vi "Module Loop.vi"(8 "error in (no error)":errorcluster, 11 "ValveControlModule in":refnum<class "ValveControlModule.lvclass">) -> (0 "error out":errorcluster, 3 "ValveControlModule out":refnum<class "ValveControlModule.lvclass">)   [LabVIEW 2020, in "VolatusControl.lvlib" / "ValveControlModule.lvclass"]
uses:
  ValveControlModule.lvclass
  C:/dev/lv20CE/relink/lv-volatus/Volatus/Module/Module.lvclass
  Volatus/Module/Module.lvclass
  Volatus/Module/Module.lvclass/Module.ctl
  messages/CmdDigital/Class/Msg.lvclass
  C:/dev/lv20CE/relink/lv-protoc/LV-Proto/Message/Message.lvclass
  messages/CmdDigital/Class/Msg.lvclass/Msg.ctl
  Volatus/MessageQ/MessageQ.lvclass/MessageQ.ctl
  messages/CmdDigital/Data.ctl
  ValveControlModule.lvclass/ValveControlModule.ctl
  messages/CmdDigitalMultiple/Data.ctl
  messages/CmdAnalog/Class/Msg.lvclass
  messages/CmdAnalog/Class/Msg.lvclass/Msg.ctl
  messages/CmdAnalog/Data.ctl
  Volatus/Module/Self Q.vi
  Volatus/MessageQ/Send.vi
  lv-vecto/Vecto/Group/Group.lvclass
  C:/dev/lv20CE/relink/lv-vecto/Vecto/GroupAbstract/GroupAbstract.lvclass
  Valve/ValveControl.lvclass
  messages/CmdDigital/CmdDigital.lvlib
  messages/CmdDigitalMultiple/CmdDigitalMultiple.lvlib
  messages/CmdAnalog/CmdAnalog.lvlib
  lv-vecto/Vecto/GroupAbstract/GroupAbstract.lvclass
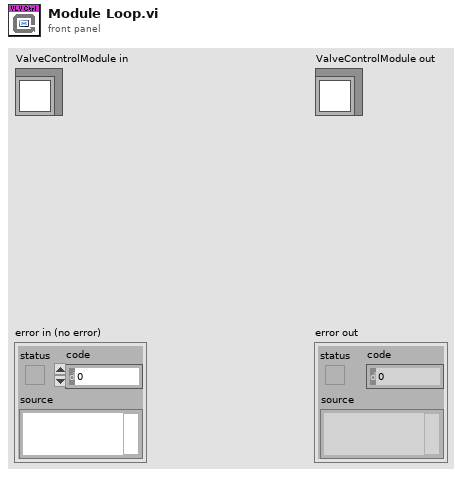
[diagram p1: front panel]
types:
  T1 = typedef "CmdDigital.lvlib/Data.ctl" = cluster{"channel":string, "value":bool}
  T2 = typedef "CmdDigitalMultiple.lvlib/Data.ctl" = cluster{"values":T1[]}
  T3 = typedef "CmdAnalog.lvlib/Data.ctl" = cluster{"channel":string, "value":dbl}
  T4 = map{string, refnum<class "ValveControl.lvclass">}
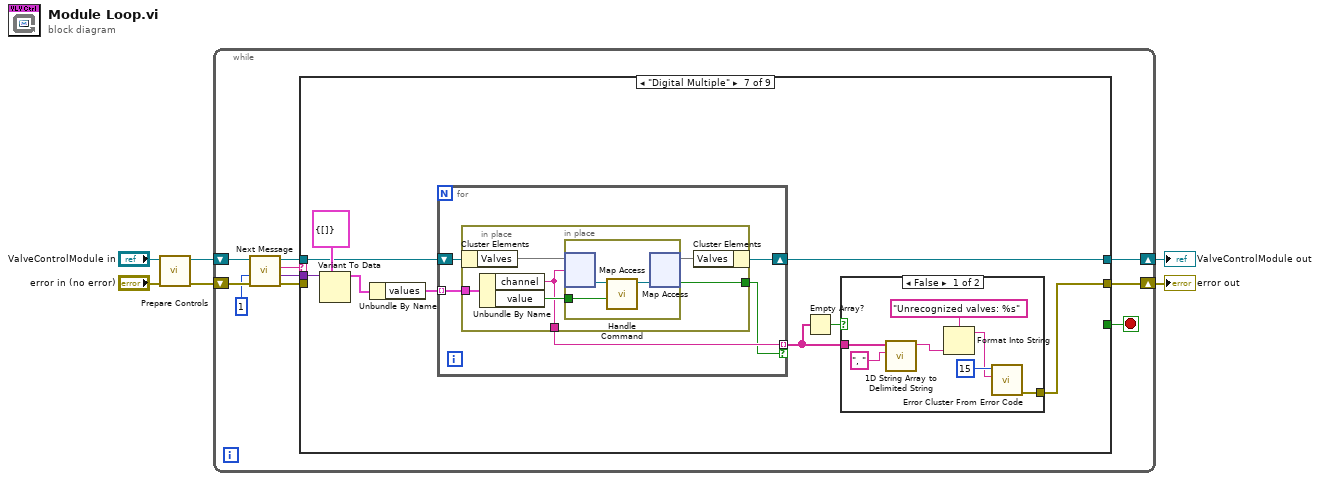
[diagram p0: block diagram]
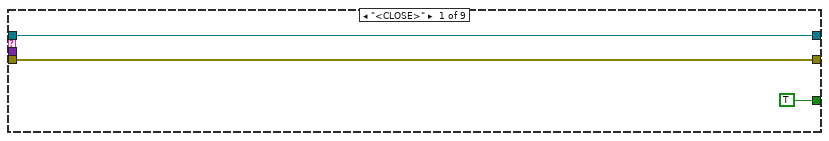
[diagram p2: hidden frame]
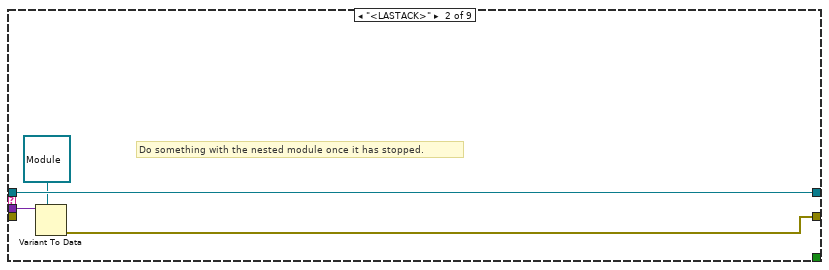
[diagram p3: hidden frame]
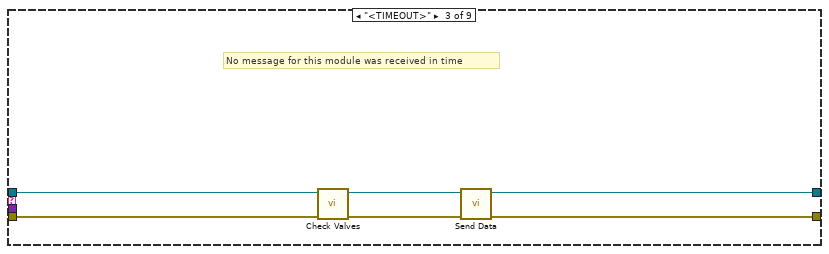
[diagram p4: hidden frame]
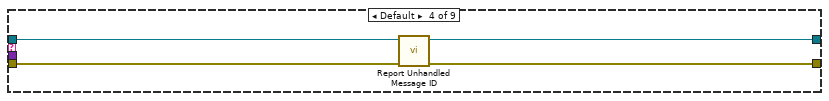
[diagram p5: hidden frame]
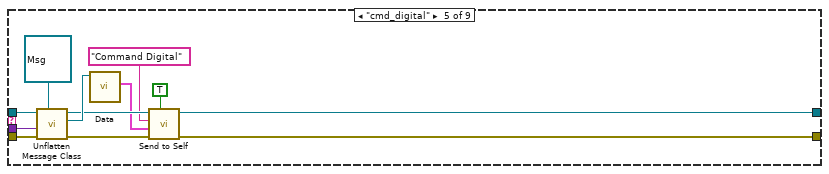
[diagram p6: hidden frame]
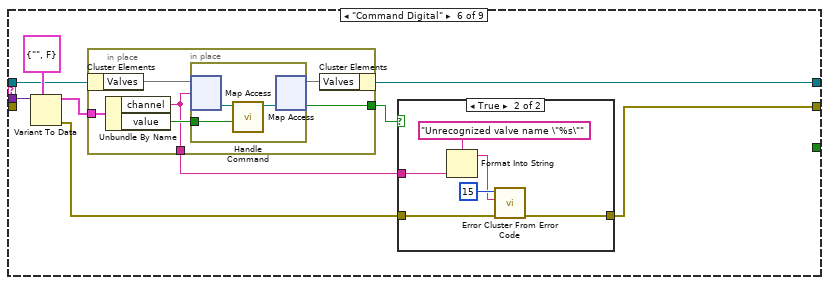
[diagram p7: hidden frame]
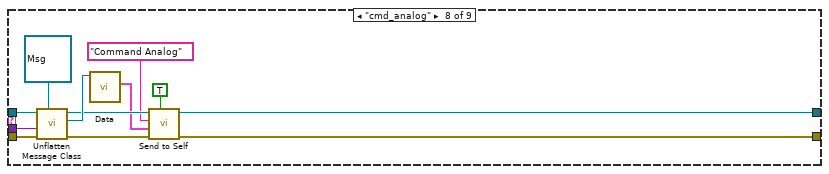
[diagram p10: hidden frame]
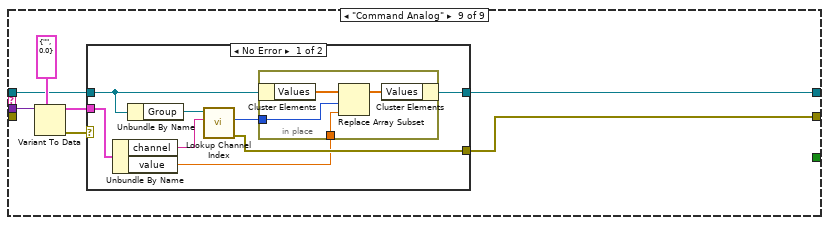
[diagram p11: hidden frame]
diagram:
  n1 = call "Prepare Controls.vi"("error in (no error)"="error in (no error)", "ValveControlModule in"="ValveControlModule in") -> ("error out"=w3:errorcluster, "ValveControlModule out"=w1:refnum<class "ValveControlModule.lvclass">)  [unwired: 8 in]
  n2 = while {
    shift-right: [w11] -> w5
    shift-left: w1 -> [w16]
    shift-right: [w10] -> w4
    shift-left: w3 -> [w15]
    stop <- w9 stop-if-true
    n3 = call "Next Message.vi"("error in (no error)"=w15, "Timeout ms (-1)"=1, "Module in"=w16) -> ("error out"=w14:errorcluster, "Data"=w8:variant, "ID"=w13:string, "Module out"=w12:refnum<class "ValveControlModule.lvclass">)  [unwired: 5 in]
    n4 = case shown="\"Digital Multiple\"" w13 {
      tunnel: w14 -> [w17 _ w29 w33 w44 _ _ w111 _]
      tunnel: w12 -> [w18 w23 w27 w31 w45 w52 w77 w112 w115]
      tunnel: [w18 w23 w24 w30 w36 w50 w76 w103 w113] -> w11
      tunnel: [w17 w20 w26 w32 w34 w46 w75 w101 w114] -> w10
      tunnel: [TRUE _ _ _ _ _ _ _ _] -> w9
      tunnel: w8 -> [_ w22 _ _ w43 w54 w79 w110 w119]
      frame "<CLOSE>" {
      }
      frame "<LASTACK>" {
        # "Do something with the nested module once it has stopped."
        n5 = Variant To Data(type=refnum<class "Module.lvclass"> refnum ("Volatus:Module"), Variant=w22) -> (error out=w20:errorcluster)  [unwired: 1 in, 1 out]
      }
      frame "<TIMEOUT>" {
        # "No message for this module was received in time"
        n6 = call "Check Valves.vi"("error in (no error)"=w29, "ValveControlModule in"=w27) -> ("error out"=w28:errorcluster, "ValveControlModule out"=w25:refnum<class "ValveControlModule.lvclass">)  [unwired: 8 in]
        n7 = call "Send Data.vi"("error in (no error)"=w28, "ValveControlModule in"=w25) -> ("error out"=w26:errorcluster, "ValveControlModule out"=w24:refnum<class "ValveControlModule.lvclass">)  [unwired: 8 in]
      }
      frame Default {
        n8 = call "Report Unhandled Message ID.vi"("error in (no error)"=w33, "Module in"=w31) -> ("error out"=w32:errorcluster, "Module out"=w30:refnum<class "ValveControlModule.lvclass">)  [unwired: 8 in]
      }
      frame "cmd_digital" {
        n9 = call "Unflatten Message Class.vi"("Message Type"=refnum<class "Msg.lvclass"> refnum ("CmdDigital.lvlib:Msg.lvclass"), "error in (no error)"=w44, "Data"=w43, "Module in"=w45) -> ("error out"=w39:errorcluster, "Message"=w41:refnum<class "Msg.lvclass">, "Module out"=w40:refnum<class "ValveControlModule.lvclass">)  [unwired: 4 in, 1 out]
        n10 = call "Data.vi"("PB Msg Template in"=w41) -> ("Data"=w37:T1)  [unwired: 8 in, 2 out]
        n11 = call "Send to Self.vi"("High Priority (F)"=TRUE, "error in (no error)"=w39, "Data"=w37, "Message ID"="Command Digital", "Module in"=w40) -> ("error out"=w34:errorcluster, "Module out"=w36:refnum<class "ValveControlModule.lvclass">)  [unwired: 5 in]
      }
      frame "Command Digital" {
        n12 = Variant To Data(type=T1 {"channel"="", "value"=FALSE} ("CmdDigital"), Variant=w54) -> (data=w51:T1, error out=w47:errorcluster)  [unwired: 1 in]
        n13 = in-place {
          in-place-border: w51 -> [w67]
          in-place-border: [w63] -> w49
          in-place-border: [w62] -> w48
          n14 = in-place-cluster #1(w52) -> ("Valves"=w66:T4)
          n15 = Unbundle By Name(w67) -> ("channel"=w62:string, "value"=w65:bool)
          n16 = in-place {
            in-place-border: w65 -> [w69]
            n17 = in-place-map #2(w66, w62) -> (w70:refnum<class "ValveControl.lvclass">)  [unwired: 1 in, 1 out]
            n18 = call-dynamic "Handle Command.vi"("Value"=w69, "Valve in"=w70) -> ("Valve out"=w68:refnum<class "ValveControl.lvclass">)  [unwired: 8 in, 1 out]
            n19 = in-place-map #2(w68) -> (w64:T4, w63:bool)  [unwired: 1 in, 1 out]
          }
          n20 = in-place-cluster #1("Valves"=w64) -> (w50:refnum<class "ValveControlModule.lvclass">)
        }
        n21 = case shown="True" w49 {
          tunnel: w48 -> [_ w61]
          tunnel: w47 -> [w55 w57]
          tunnel: [w55 w56] -> w46
          frame False {
          }
          frame True {
            n22 = Format Into String(format string="Unrecognized valve name \"%s\"", w61) -> (resulting string=w58:string)  [unwired: 2 in, 1 out]
            n23 = call <vilib>:"Error Cluster From Error Code.vi"("error in (no error)"=w57, "error message (\"\")"=w58, "error code (0)"=15) -> ("error out"=w56:errorcluster)  [unwired: 6 in]
          }
        }
      }
      frame "Digital Multiple" {
        n24 = Variant To Data(type=T2 {"values"=[]} ("CmdDigitalMultiple"), Variant=w79) -> (data=w74:T2)  [unwired: 1 in, 1 out]
        n25 = Unbundle By Name(w74) -> ("values"=w73:T1[])
        n26 = for {
          shift-right: [w83] -> w76
          shift-left: w77 -> [w84]
          tunnel: w73 -> [w82] mode=indexing
          tunnel: [w81] -> w71 mode=indexing if=w80
          n27 = in-place {
            in-place-border: [w87] -> w80
            in-place-border: [w85] -> w81
            in-place-border: w82 -> [w86]
            n28 = in-place-cluster #3(w84) -> ("Valves"=w90:T4)
            n29 = Unbundle By Name(w86) -> ("channel"=w85:string, "value"=w89:bool)
            n30 = in-place {
              in-place-border: w89 -> [w91]
              n31 = in-place-map #4(w90, w85) -> (w93:refnum<class "ValveControl.lvclass">)  [unwired: 1 in, 1 out]
              n32 = call-dynamic "Handle Command.vi"("Value"=w91, "Valve in"=w93) -> ("Valve out"=w92:refnum<class "ValveControl.lvclass">)  [unwired: 8 in, 1 out]
              n33 = in-place-map #4(w92) -> (w88:T4, w87:bool)  [unwired: 1 in, 1 out]
            }
            n34 = in-place-cluster #3("Valves"=w88) -> (w83:refnum<class "ValveControlModule.lvclass">)
          }
        }
        n35 = Empty Array?(array=w71) -> (empty?=w72:bool)
        n36 = case shown="False" w72 {
          tunnel: [w97 _] -> w75
          tunnel: w71 -> [w96 _]
          frame False {
            n37 = call <vilib>:"1D String Array to Delimited String.vi"("delimiter"=", ", "string array"=w96) -> ("delimited string"=w94:string)  [unwired: 9 in]
            n38 = Format Into String(format string="Unrecognized valves: %s", w94) -> (resulting string=w98:string)  [unwired: 2 in, 1 out]
            n39 = call <vilib>:"Error Cluster From Error Code.vi"("error message (\"\")"=w98, "error code (0)"=15) -> ("error out"=w97:errorcluster)  [unwired: 7 in]
          }
          frame True {
          }
        }
      }
      frame "cmd_analog" {
        n40 = call "Unflatten Message Class.vi"("Message Type"=refnum<class "Msg.lvclass"> refnum ("CmdAnalog.lvlib:Msg.lvclass"), "error in (no error)"=w111, "Data"=w110, "Module in"=w112) -> ("error out"=w106:errorcluster, "Message"=w108:refnum<class "Msg.lvclass">, "Module out"=w107:refnum<class "ValveControlModule.lvclass">)  [unwired: 4 in, 1 out]
        n41 = call "Data.vi"("PB Msg Template in"=w108) -> ("Data"=w104:T3)  [unwired: 8 in, 2 out]
        n42 = call "Send to Self.vi"("High Priority (F)"=TRUE, "error in (no error)"=w106, "Data"=w104, "Message ID"="Command Analog", "Module in"=w107) -> ("error out"=w101:errorcluster, "Module out"=w103:refnum<class "ValveControlModule.lvclass">)  [unwired: 5 in]
      }
      frame "Command Analog" {
        n43 = Variant To Data(type=T3 {"channel"="", "value"=0.0} ("CmdAnalog"), Variant=w119) -> (data=w116:T3, error out=w117:errorcluster)  [unwired: 1 in]
        n44 = case shown="No Error" w117 {
          selector: w117 -> [_ w133]
          tunnel: w116 -> [w126 _]
          tunnel: w115 -> [w123 w132]
          tunnel: [w127 w133] -> w114
          tunnel: [w120 w132] -> w113
          frame No Error {
            n45 = Unbundle By Name(w126) -> ("channel"=w124:string, "value"=w121:dbl)
            n46 = Unbundle By Name(w123) -> ("Group"=w125:refnum<class "Group.lvclass">)
            n47 = call "Lookup Channel Index.vi"("Channel Name"=w124, "GroupAbstract in"=w125) -> ("error out"=w127:errorcluster, "Index"=w122:i32)  [unwired: 7 in, 1 out]
            n48 = in-place {
              in-place-border: w122 -> [w130]
              in-place-border: w121 -> [w129]
              n49 = in-place-cluster #5(w123) -> ("Values"=w131:dbl[])
              n50 = Replace Array Subset(array=w131, new element=w129, index=w130) -> (w128:dbl[])
              n51 = in-place-cluster #5("Values"=w128) -> (w120:refnum<class "ValveControlModule.lvclass">)
            }
          }
          frame Error {
          }
        }
      }
    }
  }
  "error out" <- w4
  "ValveControlModule out" <- w5
